vi "VL Type.vi"(8 "error in (no error)":errorcluster, 11 "Cluster in":refnum<class "Cluster Config.lvclass">) -> (0 "error out":errorcluster, 2 "VL Type":T1, 3 "Cluster out":refnum<class "Cluster Config.lvclass">)   [LabVIEW 2020, in "VolatusConfig.lvlib" / "Cluster Config.lvclass"]
uses:
  Cluster Config.lvclass
  Meta Type.ctl
  Cluster Config.lvclass/Cluster Config.ctl
  VolatusConfig.lvlib
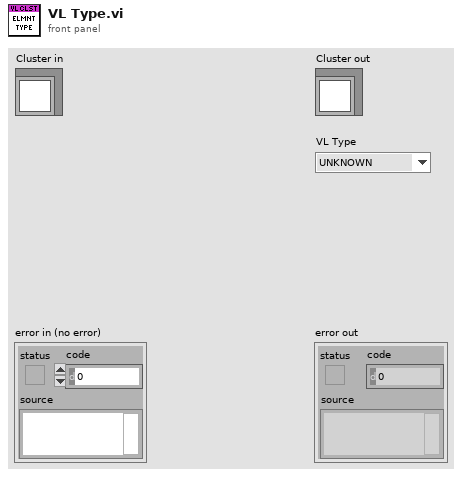
[diagram p1: front panel]
types:
  T1 = typedef "VolatusConfig.lvlib/Meta Type.ctl" = enum16{"UNKNOWN", "VL_System", "VL_Cluster", "VL_Node", "VL_Task", "VL_Group", "VL_Channel", "VL_Task_List", "VL_Scaling", "VL_Sensor", "VL_Sensor_List", "VL_Scale"}
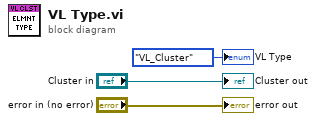
[diagram p0: block diagram]
diagram:
  "error out" <- "error in (no error)"
  "Cluster out" <- "Cluster in"
  "VL Type" <- Meta_Type."VL_Cluster" ("VL Type")
